vi "about get folder size.vi"(8 "error in (no error)":errorcluster, 11 "Directory Path":path=path "C:/") -> (0 "error out":errorcluster, 3 "Disk Space Used (MB)":dbl format="%.2f")   [LabVIEW 2011]
doc: "This VI calculates the size/disk space taken up by files in any directory and all of its subdirectories. This VI was created using LabVIEW 6.1"
panel:
  out "Calculating Size of Folder":path
  # "This VI calculates the amount of disk space used by the \nfiles in the specified folder and all of its sub-folders."
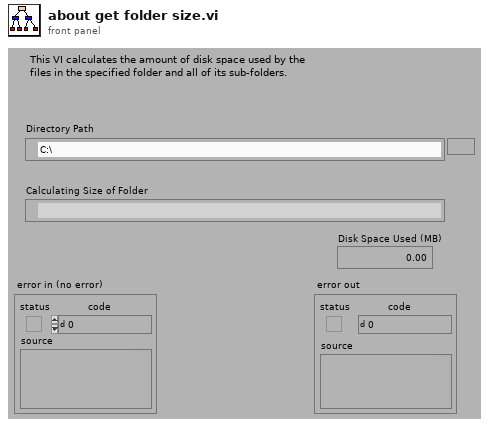
[diagram p1: front panel]
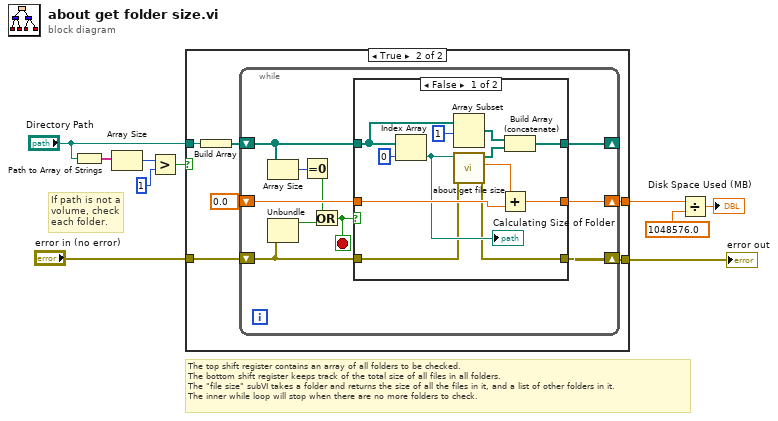
[diagram p0: block diagram]
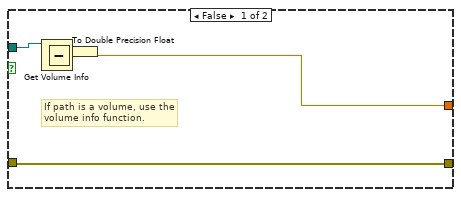
[diagram p2: hidden frame]
diagram:
  # "The top shift register contains an array of all folders to be checked.\nThe bottom shift register keeps track of the total size of all files in all folders.\nThe \"file size\" subVI takes a folder and returns the size of all the files in it, and a list of other folders in it.\nThe inner while loop will stop when there are no more folders to check."
  # "If path is not a\nvolume, check\neach folder."
  n1 = Path to Array of Strings(0:"Directory Path") -> (2:w10:string[])  [unwired: 1 out]
  n2 = Array Size(array=w10) -> (size(s)=w9:i32)
  n3 = Greater?(x=w9, y=1) -> (0:w7:bool)
  n4 = case shown="True" w7 {
    tunnel: "Directory Path" -> [w15 w22]
    tunnel: [w16 w19] -> w6
    tunnel: "error in (no error)" -> [w14 w18]
    tunnel: [w14 w17] -> w1
    frame False {
      # "If path is a volume, use the\nvolume info function."
      n5 = Get Volume Info(11:w15) -> (1:w12:i64, 2:w11:i64)  [unwired: 1 in, 4 out]
      n6 = To Double Precision Float(number=w11) -> (double precision float=w13:dbl)
      n7 = Subtract(x=w13, y=w12) -> (x-y=w16:dbl)
    }
    frame True {
      n8 = Build Array(w22) -> (w21:path[])
      n9 = while {
        shift-right: [w31] -> _
        shift-left: w21 -> [w28]
        shift-right: [w30] -> w19
        shift-left: 0.0 -> [w29]
        shift-right: [w23] -> w17
        shift-left: w18 -> [w24]
        stop <- w25 stop-if-true
        n10 = Array Size(array=w28) -> (size(s)=w32:i32)
        n11 = Unbundle(w24) -> ("status"=w27:bool)  [unwired: 2 out]
        n12 = Equal To 0?(x=w32) -> (x = 0?=w26:bool)
        n13 = Or(x=w26, y=w27) -> (x .or. y?=w25:bool)
        n14 = case shown="False" w25 {
          tunnel: [w42 w47] -> w31
          tunnel: [w40 w46] -> w30
          tunnel: w29 -> [w39 w46]
          tunnel: w28 -> [w38 w47]
          tunnel: w24 -> [w35 w45]
          tunnel: [w33 w45] -> w23
          frame False {
            n15 = Index Array(array=w38, index=0 ("length")) -> (element=w36:path)
            "Calculating Size of Folder" <- w36
            n16 = Array Subset(array=w38, index=1) -> (w43:path[])  [unwired: 1 in]
            n17 = call "about get file size.vi"("error in (no error)"=w35, "directory path"=w36) -> ("error out"=w33:errorcluster, "size"=w34:dbl, "subdir_path"=w41:path[])  [unwired: 7 in]
            n18 = Add(x=w34, y=w39) -> (x+y=w40:dbl)
            n19 = Build Array (concatenate)(w43, w41) -> (w42:path[])
          }
          frame True {
          }
        }
      }
    }
  }
  "error out" <- w1
  n20 = Divide(x=w6, y=1048576.0) -> (x/y=→"Disk Space Used (MB)":dbl)
